vi "TDT-Stream DI.vi"(0 "#Inputs":i32, 2 "Action":T1=enum."Read", 7 "Pts Per Read":i32, 11 "error in (no error)":errorcluster, 12 "DI Channels":i32[](array[numeric])=[1, 2]) -> (10 "DI Waveforms":dbl[][](array[numeric]), 15 "error out":errorcluster)   [LabVIEW 2020]
uses:
  TDT-Signal Bank Action.ctl
  TDT-Globals.vi
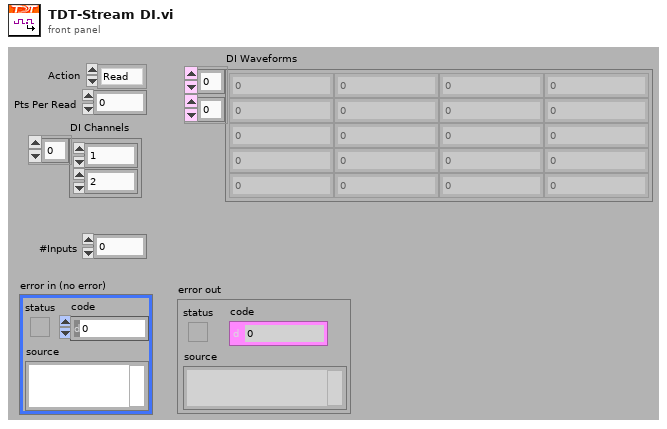
[diagram p1: front panel]
types:
  T1 = typedef "TDT-Signal Bank Action.ctl" = enum16{"Init", "Write", "Read", "Rewrite", "Reset", "Recycle", "Ramp up", "Ramp down", "Zero"}
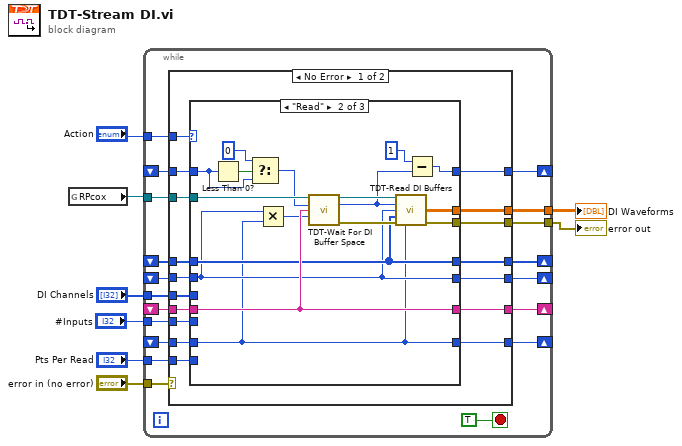
[diagram p0: block diagram]
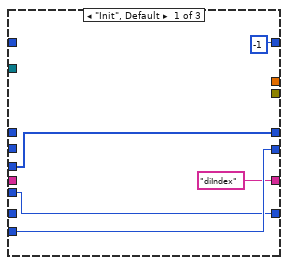
[diagram p2: hidden frame]
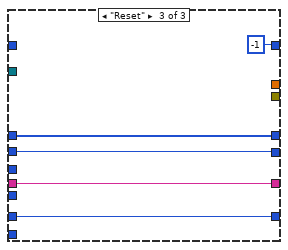
[diagram p3: hidden frame]
diagram:
  n1 = global read "TDT-Globals.vi" "RPcox"() -> (w6:refnum<k7>)
  n2 = while {
    tunnel: [w27] -> w7
    tunnel: "error in (no error)" -> [w26]
    tunnel: w6 -> [w25]
    tunnel: "Action" -> [w24]
    shift-right: [w22] -> _
    shift-left: _ -> [w21]
    tunnel: "Pts Per Read" -> [w20]
    shift-right: [w19] -> _
    shift-left: _ -> [w18]
    tunnel: [w17] -> w3
    tunnel: "DI Channels" -> [w16]
    shift-right: [w15] -> _
    shift-left: _ -> [w14]
    shift-right: [w13] -> _
    shift-left: _ -> [w12]
    shift-right: [w10] -> _
    shift-left: _ -> [w11]
    tunnel: "#Inputs" -> [w9]
    stop <- TRUE stop-if-true
    n3 = case shown="No Error" w26 {
      selector: w26 -> [_ w77]
      tunnel: [w40 w77] -> w27
      tunnel: w25 -> [w41 _]
      tunnel: w24 -> [w44 _]
      tunnel: [w43 w76] -> w22
      tunnel: w21 -> [w42 w76]
      tunnel: w20 -> [w39 _]
      tunnel: [w38 w75] -> w19
      tunnel: w18 -> [w37 w75]
      tunnel: [w36 _] -> w17
      tunnel: w16 -> [w35 _]
      tunnel: [w34 w74] -> w15
      tunnel: w14 -> [w33 w74]
      tunnel: [w32 w73] -> w13
      tunnel: w12 -> [w31 w73]
      tunnel: w11 -> [w30 w72]
      tunnel: [w29 w72] -> w10
      tunnel: w9 -> [w28 _]
      frame No Error {
        n4 = case shown="\"Read\"" w44 {
          tunnel: [-1 w66 -1] -> w43
          tunnel: w42 -> [_ w57 _]
          tunnel: w41 -> [_ w63 _]
          tunnel: [_ w61 _] -> w40
          tunnel: w39 -> [w48 _ _]
          tunnel: [w48 w51 w70] -> w38
          tunnel: w37 -> [_ w51 w70]
          tunnel: [_ w59 _] -> w36
          tunnel: w35 -> [w47 _ _]
          tunnel: [w47 w52 w71] -> w34
          tunnel: w33 -> [_ w52 w71]
          tunnel: ["diIndex" ("format string") w54 w69] -> w32
          tunnel: w31 -> [_ w54 w69]
          tunnel: w30 -> [_ w50 w67]
          tunnel: [w45 w50 w67] -> w29
          tunnel: w28 -> [w45 _ _]
          frame "Init", Default {
          }
          frame "Read" {
            n5 = Less Than 0?(x=w57) -> (x < 0?=w58:bool)
            n6 = Select(t=0, s=w58, f=w57) -> (s? t:f=w55:i32)
            n7 = Multiply(x=w51, y=w50) -> (x*y=w53:i32)
            n8 = call "TDT-Wait For DI Buffer Space.vi"("RPcox"=w63, "Next Buffer"=w55, "Tag"=w54, "Buffer Length"=w53) -> ("RPcox Out"=w62:refnum<k7>, "Next Buffer Out"=w60:i32, "error out"=w64:errorcluster)  [unwired: 9 in]
            n9 = call "TDT-Read DI Buffers.vi"("RPcox"=w62, "Next Buffer"=w60, "Pts Per Read"=w51, "DI Channels"=w52, "error in (no error)"=w64, "#inputs"=w50) -> ("Input array"=w59:dbl[][], "error out"=w61:errorcluster)  [unwired: 8 in]
            n10 = Subtract(x=1, y=w60) -> (x-y=w66:i32)
          }
          frame "Reset" {
          }
        }
      }
      frame Error {
      }
    }
  }
  "error out" <- w7
  "DI Waveforms" <- w3
